vi "Simple Wireless Logging.vi"() -> ()   [LabVIEW 2018]
uses:
  ff44e4a9-c346-414c-ae2a-efcf3ff82913.vi
  src/api/logger_class/Logger.lvclass
  src/api/Log Levels.ctl
  src/api/GLog.lvlib
  19e8f962-4a22-47f2-af30-cb2bfea6a4c8.vi
  d05347f3-4e1b-46da-8a6f-00907147f5e9.vi
  985cbf90-cda4-43bb-963b-ba8b8541f322.vi
panel:
  out "ms timer":u32[](array[numeric])
  out "elapsed time":u32[](array[numeric])
  out "iterations":i32[](array[numeric])
  in  "error in (no error)":errorcluster
  out "error out":errorcluster
  in  "total iterations":i32=30
  # "Locals"
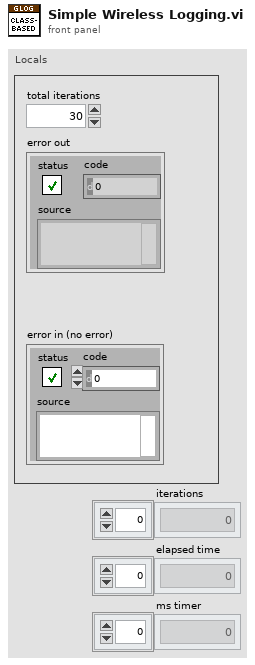
[diagram p1: front panel]
types:
  T1 = typedef "GLog.lvlib/Log Levels.ctl" = enum16{"Trace", "Debug", "Info", "Warning", "Error", "Critical"}
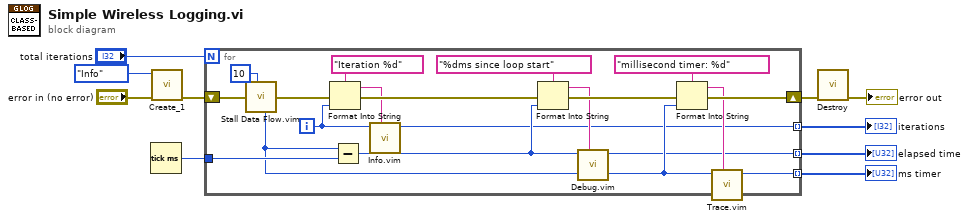
[diagram p0: block diagram]
diagram:
  n1 = Tick Count (ms)() -> (millisecond timer value=w10:u32)
  n2 = call "Create_1.vi"("error in (no error)"="error in (no error)", "minimum log level (Info)"=Log_Levels."Info" ("minimum log level")) -> ("error out"=w6:errorcluster)  [unwired: 9 in]
  n3 = for {
    N: "total iterations" -> [_]
    tunnel: w10 -> [w29]
    shift-right: [w22] -> w5
    shift-left: w6 -> [w15]
    tunnel: [w13] -> w3 mode=indexing
    tunnel: [w12] -> w2 mode=indexing
    tunnel: [w11] -> w1 mode=indexing
    i -> [w21]
    n4 = call "Stall Data Flow.vim"("value in"=w15, "milliseconds to wait"=u32 10 ("loop iteration delay [ms]")) -> ("millisecond timer value"=w17:u32, "value out"=w14:errorcluster)
    n5 = Format Into String(format string="Iteration %d" ("message"), error in=w14, w21) -> (resulting string=w20:string, error out=w24:errorcluster)  [unwired: 1 in]
    n6 = Subtract(x=w17, y=w29) -> (x-y=w18:u32)
    n7 = call "Info.vim"("data in (null)"=w21, "message"=w20) -> ("data out"=w13:i32)  [unwired: 9 in]
    n8 = Format Into String(format string="%dms since loop start" ("message"), error in=w24, w18) -> (resulting string=w19:string, error out=w23:errorcluster)  [unwired: 1 in]
    n9 = call "Debug.vim"("data in (null)"=w18, "message"=w19) -> ("data out"=w12:u32)  [unwired: 9 in]
    n10 = Format Into String(format string="millisecond timer: %d" ("message"), error in=w23, w17) -> (resulting string=w16:string, error out=w22:errorcluster)  [unwired: 1 in]
    n11 = call "Trace.vim"("data in (null)"=w17, "message"=w16) -> ("data out"=w11:u32)  [unwired: 9 in]
  }
  "iterations" <- w3
  "elapsed time" <- w2
  "ms timer" <- w1
  n12 = call "Destroy.vi"("error in (no error)"=w5) -> ("error out"=→"error out":errorcluster)  [unwired: 9 in, 1 out]
